vi "Shutdown.vi"(8 "error in (no error)":errorcluster) -> (0 "error out":errorcluster)   [LabVIEW 2025, in "Logitech Devices.lvlib"]
uses:
  Logitech Devices.lvlib
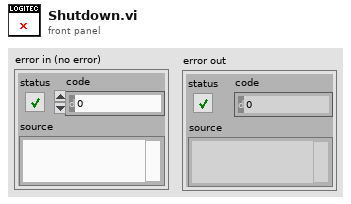
[diagram p1: front panel]
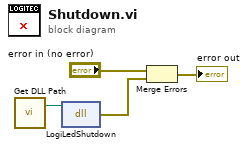
[diagram p0: block diagram]
diagram:
  n1 = call "Get DLL Path.vi"() -> ("LG Hub SDK DLL"=w1:path)  [unwired: 3 in]
  n2 = dll-call lib="C:/Program Files/LGHUB/sdks/sdk_legacy_led_x86.dll" fn="LogiLedShutdown"(path in=w1) -> (error out=w2:errorcluster)  [unwired: 3 in, 1 out]
  n3 = Merge Errors("error in (no error)", w2) -> (→"error out":errorcluster)
